vi "Check Valid Message.vi"(8 "error in (no error)":errorcluster, 10 "Message":string, 11 "Pump Controller in":refnum<class "Pump Controller.lvclass">) -> (0 "error out":errorcluster, 2 "Valid?":bool, 3 "Pump Controller out":refnum<class "Pump Controller.lvclass">)   [LabVIEW 2020, in "Pump Controller.lvclass"]
uses:
  Pump Controller.lvclass
  Pump Controller.lvclass/Pump Controller.ctl
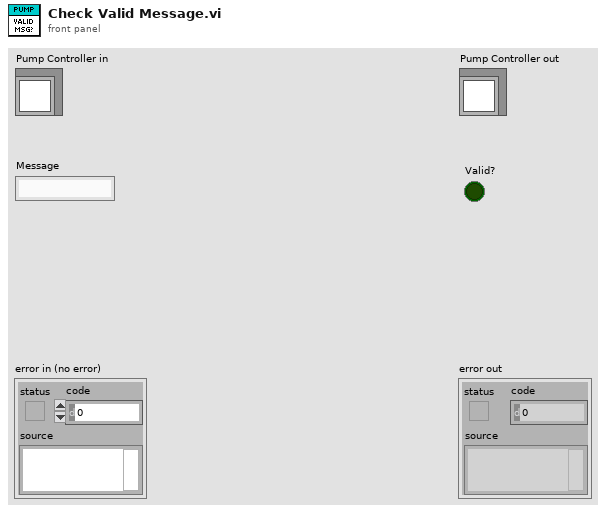
[diagram p1: front panel]
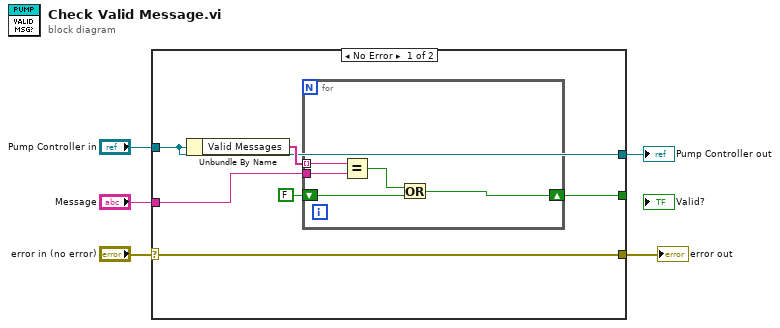
[diagram p0: block diagram]
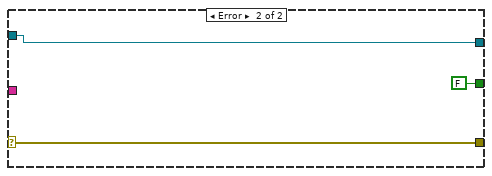
[diagram p2: hidden frame]
diagram:
  n1 = case shown="No Error" "error in (no error)" {
    selector: "error in (no error)" -> [w8 w18]
    tunnel: [w11 FALSE ("Valid?")] -> _
    tunnel: "Pump Controller in" -> [w7 w19]
    tunnel: "Message" -> [w10 _]
    tunnel: [w8 w18] -> w4
    tunnel: [w7 w19] -> w1
    frame No Error {
      n2 = Unbundle By Name(w7) -> ("Valid Messages"=w9:string[])
      n3 = for {
        tunnel: w9 -> [w15] mode=indexing
        tunnel: w10 -> [w16]
        shift-right: [w12] -> w11
        shift-left: FALSE -> [w13]
        n4 = Equal?(x=w15, y=w16) -> (x = y?=w14:bool)
        n5 = Or(x=w14, y=w13) -> (x .or. y?=w12:bool)
      }
    }
    frame Error {
    }
  }
  "error out" <- w4
  "Pump Controller out" <- w1
